vi "Audio Plugin UI Meas Ser1 - multichannel.vi"() -> ()   [LabVIEW 2021]
uses:
  <vilib>/PDM Acquisition Toolkit/shared/controls/i2s frame size.ctl
  <vilib>/PDM Acquisition Toolkit/host/Classes/Tasks/PDM Tasks/Controls/Acquisition Mode.ctl
  <vilib>/addons/_NISVFA/_Shared subVIs/Controls/svc_Window.ctl
  <vilib>/addons/_NISVFA/_Shared subVIs/Common/SVL Set dB Reference (N Ch - 1 Ref).vi
  <vilib>/addons/Sound and Vibration/svt_Level/SVL AC & DC Level (Time) (N Ch).vi
  <vilib>/addons/Sound and Vibration/svt_Single Tone Measurements/SVT Spurious Free Dynamic Range (Frequency) (1 Ch).vi
  <vilib>/addons/_NISVFA/_Shared subVIs/Common/SVL Set dB Reference (1 Ch).vi
  <vilib>/addons/Sound and Vibration/svt_Level/SVL AC & DC Level (Time) (1 Ch).vi
  <vilib>/addons/_NISVFA/_Spectrum Processing/SVFA Get Spectrum Subset.vi
  <vilib>/addons/_NISVFA/_Spectrum Processing/SVFA Get Spectrum Subset (Complex) (1 Ch).vi
  <vilib>/addons/_NISVFA/_Shared subVIs/Common/svc_Window Parameters.vi
  <vilib>/addons/_NISVFA/_Shared subVIs/Common/svc_Extract Single Tone Information (complex).vi
  <vilib>/addons/_NISVFA/_Shared subVIs/Common/svc_Check Frequency Range in Spectrum.vi
  <vilib>/addons/_NISVFA/_Spectrum Processing/SVFA Unit Conversion.vi
  <vilib>/addons/_NISVFA/_Spectrum Processing/SVFA Unit Conversion (Complex) (1 Ch).vi
  <vilib>/addons/_NISVFA/_Spectrum Processing/SVFA Spectrum Peak Search.vi
  <vilib>/addons/_NISVFA/_Spectrum Processing/SVFA Spectrum Peak Search (1 Ch).vi
  <vilib>/addons/_NISVFA/_Shared subVIs/Common/svc_Spectrum Units.vi
  <vilib>/addons/_NISVFA/_Shared subVIs/Common/SVL Set dB Reference (variant).vi
  <vilib>/addons/_NISVFA/_Shared subVIs/Common/svc_Get SV Channel Info.vi
  <vilib>/Analysis/baseanly.llb/Mean.vi
  <vilib>/Analysis/baseanly.llb/Mean (DBL).vi
  <vilib>/addons/_NISVFA/_Shared subVIs/Windowing/svfa_Scaled Time Domain Window (Array).vi
  <vilib>/addons/_NISVFA/_Shared subVIs/Common/svc_Build Unit Label for Frequency Range.vi
  <vilib>/addons/_NISVFA/_Spectrum Processing/SVFA Get Tone Amplitude and Phase (1 Ch).vi
  <vilib>/addons/_NISVFA/_Spectrum Processing/subVIs/svfa_Compute Complex Spectrum for Export.vi
  <vilib>/addons/_NISVFA/_Shared subVIs/Common/svc_Check Frequency Range in Bandwidth.vi
  <vilib>/addons/_NISVFA/_Shared subVIs/Common/svc_Convert Start and Stop to Start Index and Length.vi
  <vilib>/addons/_NISVFA/_Shared subVIs/Common/svc_Log View for Spectrum (1Ch).vi
  <vilib>/addons/_NISVFA/_Spectrum Processing/SVFA Unit Conversion (1 Ch).vi
  <vilib>/addons/_NISVFA/_Shared subVIs/Common/svc_Complex Datatype Defaults.vi
  <vilib>/addons/_NISVFA/_Spectrum Processing/subVIs/svfa_Spectrum Peak Search.vi
  <vilib>/addons/_NISVFA/_Shared subVIs/Common/svc_Format Value (DBL).vi
  <vilib>/addons/_NISVFA/_Shared subVIs/Common/svc_Get Weighting Enum and Labels.vi
  <vilib>/addons/_NISVFA/_Shared subVIs/Common/svc_Engineering Units to Unit Label.vi
  <vilib>/addons/_NISVFA/_Shared subVIs/Common/svc_Surround NonAlpha String with Parentheses.vi
  <vilib>/dlg_ctls.llb/Space Constant.vi
  <vilib>/addons/_NISVFA/_Shared subVIs/Common/svc_Unit Label to Engineering Units.vi
  <vilib>/addons/_NISVFA/_Spectrum Processing/subVIs/svfa_Spectrum Info Window to windowTd Type Def.vi
  <vilib>/Analysis/4window.llb/Force Window.vi
  <vilib>/Analysis/4window.llb/Force Window (DBL).vi
  <vilib>/Analysis/4window.llb/Exponential Window.vi
  <vilib>/Analysis/4window.llb/Exponential Window (DBL).vi
  <vilib>/addons/_NISVFA/_Spectrum Processing/subVIs/svfa_Window Frequency Response.vi
  <vilib>/addons/_NISVFA/_Spectrum Processing/subVIs/svfa_Window Frequency Response (double array).vi
  <vilib>/Analysis/baseanly.llb/Dot Product.vi
  <vilib>/Analysis/baseanly.llb/Complex Dot Product.vi
  <vilib>/addons/_NISVFA/_Shared subVIs/Common/svc_Unwrap Phase.vi
  <vilib>/addons/_NISVFA/_Shared subVIs/Common/svc_Convert Spectrum Array to dB.vi
  <vilib>/addons/_NISVFA/_Spectrum Processing/subVIs/svfa_Conversion Utility (spectrum info).vi
  <vilib>/addons/_NISVFA/_Spectrum Processing/subVIs/svfa_Peak Rough Search Indices.vi
  <vilib>/addons/_NISVFA/_Shared subVIs/Common/svc_Unit Label Lexical Class.vi
  <vilib>/addons/_NISVFA/_Spectrum Processing/subVIs/svfa_Rect Window Frequency Response.vi
  <vilib>/addons/_NISVFA/_Spectrum Processing/subVIs/svfa_Cosine Window Coefficients.vi
  <vilib>/addons/_NISVFA/_Spectrum Processing/subVIs/svfa_Peak to RMS to Peak2Peak.vi
  <vilib>/addons/_NISVFA/_Spectrum Processing/subVIs/svfa_Mag to Mag2.vi
  <vilib>/addons/_NISVFA/_Spectrum Processing/subVIs/svfa_Linear to dB.vi
  <vilib>/addons/_NISVFA/_Spectrum Processing/subVIs/svfa_dBrefA to dBrefB.vi
  <vilib>/addons/_NISVFA/_Spectrum Processing/subVIs/svfa_Spectrum to Spectral Density.vi
  <vilib>/PDM Acquisition Toolkit/host/API/Public/Create Tasks/Create I2S Input Task.vi
  <vilib>/PDM Acquisition Toolkit/host/API/Public/Configure/Timing/Configure Timing - I2S Input Slave.vi
  <vilib>/PDM Acquisition Toolkit/host/API/Public/Configure/PDM Channel/Configure Microphone Sensitivity FSPA - I2S Input Task.vi
  <vilib>/DAQmx/create/channels.llb/DAQmx Create Channel (AO-FuncGen).vi
  <vilib>/PDM Acquisition Toolkit/host/API/Public/Commit/Commit I2S Input Task.vi
  <vilib>/PDM Acquisition Toolkit/host/API/Public/Start/Start I2S Input Task.vi
  <vilib>/PDM Acquisition Toolkit/host/API/Public/Read/Read I2S Waveform.vi
  <vilib>/PDM Acquisition Toolkit/host/API/Public/Clear/Clear I2S Input Task.vi
  <vilib>/addons/Sound and Vibration/svt_Weighting/SVT Weighting Filter (N Ch).vi
  <vilib>/addons/_NISVFA/_Shared subVIs/Common/svc_Caller VI Returned in Error Source.vi
  <vilib>/addons/_NISVFA/_Shared subVIs/Common/svc_Get Window Info.vi
  <vilib>/Analysis/0measdsp.llb/Scaled Time Domain Window.vi
  <vilib>/Analysis/0measdsp.llb/Scaled Time Domain Window (DBL).vi
  <vilib>/Utility/error.llb/Error Cluster From Error Code.vi
  <vilib>/Analysis/baseanly.llb/Std Deviation and Variance.vi
  <vilib>/addons/Sound and Vibration/svt_Single Tone Measurements/SVT Gain (Time) (1 Ch).vi
  <vilib>/addons/Sound and Vibration/svt_Distortion/SVT SNR without Harmonics (Frequency) (1 Ch).vi
  <vilib>/addons/Sound and Vibration/svt_Single Tone Measurements/SVT Dynamic Range (Frequency) (1 Ch).vi
  <vilib>/addons/Sound and Vibration/svt_Distortion/subVIs/sv_Check Data Valid (Audio) (1 Ch).vi
  <vilib>/addons/_NISVFA/_Shared subVIs/Common/svc_Convert Frequency to Frequency String.vi
  <vilib>/Analysis/4window.llb/window parameters.vi
  <vilib>/Analysis/4window.llb/Window Properties.vi
  <vilib>/Analysis/4window.llb/Window Properties by Name.vi
  <vilib>/addons/_NISVFA/_Spectrum Processing/subVIs/svfa_Spectrum Peak Tone Search and Estimation (complex).vi
  <vilib>/measure/masignal.llb/Tones and Noise Waveform.vi
  <vilib>/addons/_NISVFA/_Shared subVIs/Common/svc_FFT with Window.vi
  <vilib>/Analysis/1siggen.llb/Square Wave.vi
  <vilib>/addons/_NISVFA/_Spectrum Processing/subVIs/svfa_Three Finger Peak Search.vi
  <vilib>/addons/Sound and Vibration/svt_Distortion/subVIs/sv_Peak View Amplitude (1 Ch).vi
  <vilib>/PDM Acquisition Toolkit/host/Classes/Tasks/PDM Tasks/PDM Task.lvclass
  <vilib>/PDM Acquisition Toolkit/host/API/PDM Acquisition Toolkit.lvlib
  <vilib>/addons/Sound and Vibration/svt_Single Tone Measurements/SoundVib_SingleTone.lvlib
  <vilib>/addons/Sound and Vibration/svt_Distortion/SoundVib_Distortion.lvlib
  <vilib>/PDM Acquisition Toolkit/shared/PDM Shared.lvlib
  <vilib>/addons/Sound and Vibration/svt_Weighting/SoundVib_ABCWeighting.lvlib
panel:
  in  "Array":string[](array[string])
  in  "weighting":u16(ring) items=["Linear", "A-weighting", "B-weighting", "C-weighting"]
  in  "Bits per Sample":u32=16 caption="BITS PER SAMPLE"
  in  "DUT full scale (V pk)":dbl=3.16 format="%.3p"
  out "error out":errorcluster
  out "Sampling Rate":dbl=192000.0 format="%#_6p"
  in  "I2S Data Latch at SCK Cycle":u8=50 caption="DATA LATCH AT SCK" format="%.0f%"
  out "MeasTable":string[][](table)
  in  "I2S Logic Level":enum16{"3.3 V", "1.8 V", "1.2 V"}(ring) caption="LOGIC LEVEL"
  in  "I2S Frame Size":enum16{"32bits", "64bits"}(ring)=enum."64bits" caption="FRAME SIZE"
  in  "I2S Number of Words":u32=19200 caption="NO OF WORDS"
  in  "I2S Word Length":u32=24 caption="WORD LENGTH"
  in  "I2S Clock Rate":u32=12288000 caption="CLOCK RATE"
  in  "THD Maximum Harmonic":u32=9 caption="MAX HARMONIC"
  in  "Measurement Band Stop":dbl=20000.0 caption="BAND STOP" format="%#_6pHz"
  in  "Measurement Band Start":dbl=20.0 caption="BAND START" format="%#_6pHz"
  in  "DSG amplitude":dbl=1.0 caption="AMPLITUDE" format="%#_6pV"
  in  "DSG frequency":dbl=1000.0 caption="FREQUENCY" format="%#_6pHz"
  in  "Mic sensitivity (FS/Pa)":dbl=0.34762 caption="MIC SENSITIVITY" format="%.3fFS/Pa"
  in  "I2S Channel List":string="PXI1Slot7\\I2Si 0" caption="CHANNEL LIST"
  out "MeasGraphs":enum32{"Time Domain", "Histogram", "DNL", "INL"}(tab)
  out "TimeDomain":waveform(dbl)[](graph) caption="AC"
  # "Can we hard code Sensitivity? \nAdd weighting filter option from SV toolkit"
  # "Analog Source"
  # "Measurement"
  # "I2S Setting"
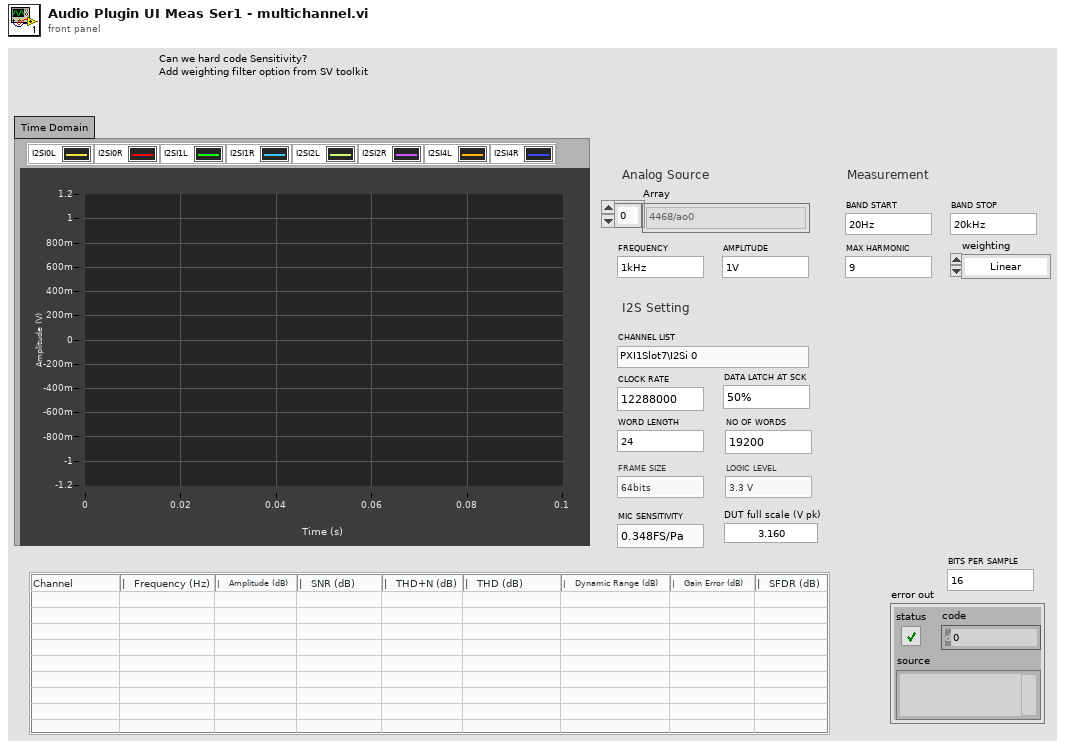
[diagram p1: front panel]
types:
  T1 = cluster{"band start (Hz)":dbl, "band stop (Hz)":dbl}
  T2 = typedef "PDM Shared.lvlib/i2s frame size.ctl" = enum16{"32bits", "64bits"}
  T3 = cluster{"frequency range":cluster{"band start (Hz)":dbl, "band stop (Hz)":dbl}, "THD maximum harmonic":i32, "amplitude":dbl, "frequency (Hz)":dbl, "microphone sensitivity (FS/Pa)":dbl, "number of words":i32, "channel list":string, "logic level":enum16{"3.3 V", "1.8 V", "1.2 V"}, "I2S serial clock rate 2":u32, "frame size":T2, "word length":u32, "Data Latch at SCK cycle":u8, "Playback .WAV File?":bool, "Record .WAV File?":bool, "Record wave file path":path, "Playback .WAV file path":path, "number of channels":i32, "DUT full scale (V pk)":dbl, "output channel":tag[]}
  T4 = typedef "PDM Acquisition Class Library.lvlib/PDM Task.lvclass/Acquisition Mode.ctl" = enum16{"Finite", "Continuous"}
  T5 = cluster{"gain units":enum16{"dB", "linear ratio"}, "detected fundamental amplitude units":enum16{"EU rms", "EU peak", "EU peak-peak"}}
  T6 = cluster{"SNR units":enum16{"dB", "linear ratio", "%"}, "detected fundamental amplitude units":enum16{"EU rms", "EU peak", "EU peak-peak"}}
  T7 = typedef "PDM Acquisition Class Library.lvlib/I2S Input Task.lvclass/DVR I2S Input Task.ctl" = refnum<data-value>
  T8 = typedef "svc_Window.ctl" = u32
  T9 = typedef "svc_Spectrum Info.ctl" = cluster{"channel name":string, "description":string, "x-axis units":T10, "spectral info":cluster{"spectrum type":T11, "linear/dB":enum16{"linear", "dB"}, "window":u16, "window size":i32, "FFT size":i32}, "engineering units":T12, "custom label":string, "dB reference [EU]":dbl, "peak units":enum16{"rms", "peak", "peak-peak"}, "weighting filter":T13, "spectral density?":bool, "unit label":string, "spectrum skewed?":bool, "complimentary spectrum units":T14}
  T10 = typedef "svc_X-Axis Units.ctl" = u16
  T11 = typedef "svc_Spectrum Type.ctl" = enum16{"FFT Spectrum [complex]", "Amplitude [Magnitude]", "Power [Magnitude^2]", "Cross Spectrum [complex]", "Frequency Response [Complex]"}
  T12 = typedef "svc_Engineering Units Text Ring.ctl" = u16
  T13 = typedef "svc_Weighting Filter Text Ring.ctl" = u16
  T14 = typedef "svc_Complimentary Spectrum Units.ctl" = enum16{"none", "radians", "degrees", "cycles", "imaginary"}
  T15 = cluster{"complex spectrum response":cluster{"f0":dbl, "df":dbl, "complex spectrum":cdb[]}, "spectrum info":T9}
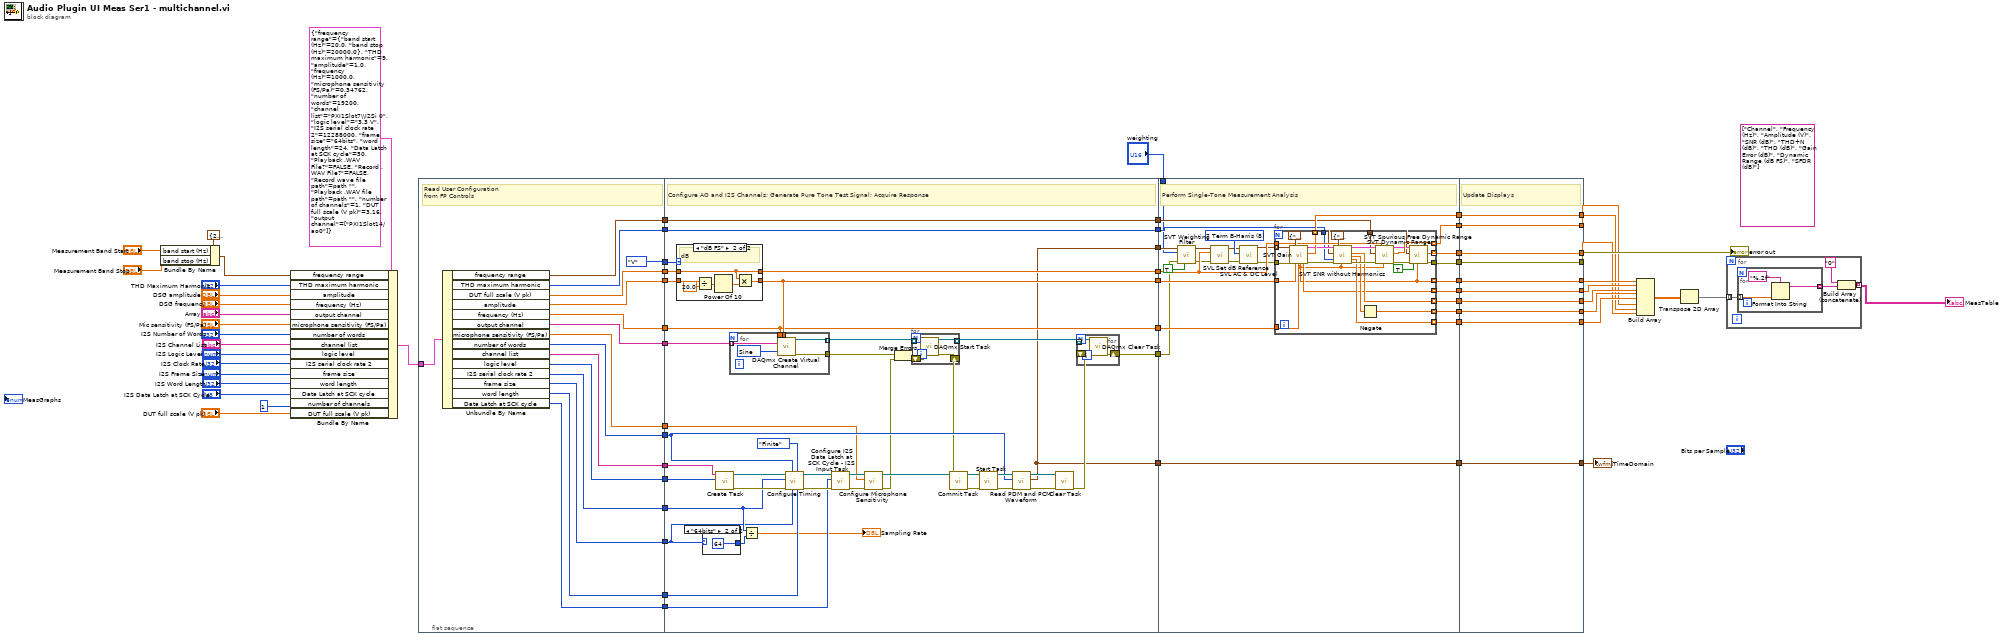
[diagram p0: block diagram]
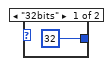
[diagram p2: hidden frame]
diagram:
  (unwired) string[] ["Channel", "Frequency (Hz)", "Amplitude (V)", "SNR (dB)", "THD+N (dB)", "THD (dB)", "Gain Error (dB)", "Dynamic Range (dB FS)", "SFDR (dB)"] ("MeasTable")
  n1 = Bundle By Name(cluster=T1 {"band start (Hz)"=20.0, "band stop (Hz)"=20000.0} ("frequency range"), "band start (Hz)"="Measurement Band Start", "band stop (Hz)"="Measurement Band Stop") -> (w33:T1)
  n2 = Bundle By Name(cluster=T3 {"frequency range"={"band start (Hz)"=20.0, "band stop (Hz)"=20000.0}, "THD maximum harmonic"=9, "amplitude"=1.0, "frequency (Hz)"=1000.0, "microphone sensitivity (FS/Pa)"=0.34762, "number of words"=19200, "channel list"="PXI1Slot7\\I2Si 0", "logic level"=enum."3.3 V", "I2S serial clock rate 2"=12288000, "frame size"=enum."64bits", "word length"=24, "Data Latch at SCK cycle"=50, "Playback .WAV File?"=FALSE, "Record .WAV File?"=FALSE, "Record wave file path"=path "", "Playback .WAV file path"=path "", "number of channels"=1, "DUT full scale (V pk)"=3.16, "output channel"=["PXI1Slot14/ao0"]}, "frequency range"=w33, "THD maximum harmonic"="THD Maximum Harmonic", "amplitude"="DSG amplitude", "frequency (Hz)"="DSG frequency", "output channel"="Array", "microphone sensitivity (FS/Pa)"="Mic sensitivity (FS/Pa)", "number of words"="I2S Number of Words", "channel list"="I2S Channel List", "logic level"="I2S Logic Level", "I2S serial clock rate 2"="I2S Clock Rate", "frame size"="I2S Frame Size", "word length"="I2S Word Length", "Data Latch at SCK cycle"="I2S Data Latch at SCK Cycle", "number of channels"=1, "DUT full scale (V pk)"="DUT full scale (V pk)") -> (w20:T3)
  n3 = flat-sequence {
    tunnel: [w80] -> w67
    tunnel: [w77] -> w66
    tunnel: [w76] -> w65
    tunnel: [w79] -> w64
    tunnel: [w78] -> w63
    tunnel: [enum16{"V", "dB FS"}."V" ("amplitude units")] -> w62
    tunnel: [w71] -> w61
    tunnel: [w72] -> w60
    tunnel: [w68] -> w59
    tunnel: [w74] -> w58
    tunnel: [w69] -> w57
    tunnel: [w70] -> w56
    tunnel: [w73] -> w55
    tunnel: [w75] -> w39
    tunnel: w20 -> [w82]
    tunnel: [w81] -> w19
    tunnel: w67 -> [w121]
    tunnel: w66 -> [w114]
    tunnel: w65 -> [w119]
    tunnel: w64 -> [w124]
    tunnel: w63 -> [w123]
    tunnel: w62 -> [w120]
    tunnel: [w125] -> w54
    tunnel: [w122] -> w53
    tunnel: [w121] -> w52
    tunnel: [w118] -> w51
    tunnel: [w114] -> w50
    tunnel: [w84] -> w49
    tunnel: [w112] -> w48
    tunnel: w61 -> [w96]
    tunnel: w60 -> [w95]
    tunnel: w59 -> [w94]
    tunnel: w58 -> [w93]
    tunnel: w57 -> [w92]
    tunnel: w56 -> [w91]
    tunnel: w55 -> [w90]
    tunnel: w39 -> [w85]
    tunnel: w19 -> [w125]
    tunnel: [w84] -> w15
    tunnel: [w169] -> w47
    tunnel: [w168] -> w46
    tunnel: [w159] -> w45
    tunnel: [w167] -> w44
    tunnel: [w166] -> w43
    tunnel: [w165] -> w42
    tunnel: [w164] -> w41
    tunnel: [w158] -> w40
    tunnel: w54 -> [w157]
    tunnel: w53 -> [w171]
    tunnel: w52 -> [w162]
    tunnel: w51 -> [w170]
    tunnel: w50 -> [w163]
    tunnel: w49 -> [w155]
    tunnel: w48 -> [w153]
    tunnel: [w160] -> w16
    tunnel: w15 -> [w160]
    tunnel: [w156] -> w14
    tunnel: "weighting" -> [w151]
    tunnel: w47 -> [w203]
    tunnel: w46 -> [w202]
    tunnel: w45 -> [w210]
    tunnel: w44 -> [w204]
    tunnel: w43 -> [w205]
    tunnel: w42 -> [w206]
    tunnel: w41 -> [w207]
    tunnel: w40 -> [w208]
    tunnel: [w210] -> w38
    tunnel: [w209] -> w17
    tunnel: w16 -> [w209]
    tunnel: w14 -> [w201]
    tunnel: [w208] -> w13
    tunnel: [w207] -> w12
    tunnel: [w206] -> w11
    tunnel: [w205] -> w10
    tunnel: [w204] -> w9
    tunnel: [w203] -> w8
    tunnel: [w202] -> w7
    tunnel: [w201] -> w6
    frame #0 {
      # "Read User Configuration\nfrom FP Controls"
      n4 = Unbundle By Name(w82) -> ("frequency range"=w81:T1, "THD maximum harmonic"=w80:i32, "DUT full scale (V pk)"=w79:dbl, "amplitude"=w78:dbl, "frequency (Hz)"=w77:dbl, "output channel"=w76:tag[], "microphone sensitivity (FS/Pa)"=w75:dbl, "number of words"=w74:i32, "channel list"=w73:string, "logic level"=w72:enum16{"3.3 V", "1.8 V", "1.2 V"}, "I2S serial clock rate 2"=w71:u32, "frame size"=w70:T2, "word length"=w69:u32, "Data Latch at SCK cycle"=w68:u8)
    }
    frame #1 {
      # "Configure AO and I2S Channels; Generate Pure Tone Test Signal; Acquire Response"
      n5 = case shown="\"dB FS\"" w120 {
        tunnel: [w142 w144] -> w118
        tunnel: w123 -> [w142 w148]
        tunnel: w124 -> [w141 w143]
        tunnel: [w141 w143] -> w122
        frame Default {
          # "V"
        }
        frame "dB FS" {
          # "dB"
          n6 = Divide(x=w148, y=20.0) -> (x/y=w146:dbl)
          n7 = Power Of 10(x=w146) -> (10^x=w145:dbl)
          n8 = Multiply(x=w143, y=w145) -> (x*y=w144:dbl)
        }
      }
      n9 = case shown="\"64bits\"" w91 {
        tunnel: [u8 32 ("frame size") u8 64 ("frame size")] -> w100
        frame "32bits" {
        }
        frame "64bits" {
        }
      }
      n10 = call-poly <vilib>:"Create Task.vi"("logic level"=w95, "channel list"=w90) -> ("error out"=w106:errorcluster, "I2S input task out"=w105:T7)  [unwired: 8 in]
      n11 = for {
        tunnel: w119 -> [w138] mode=indexing
        tunnel: w118 -> [w137]
        tunnel: [w136] -> w117
        tunnel: [w135] -> w115 mode=indexing
        tunnel: w114 -> [w134]
        w133 = 14751 items=["Sine"=14751, "Triangle"=14752, "Square"=14753, "Sawtooth"=14754] ("type")
        n12 = call-poly <vilib>:"DAQmx Create Virtual Channel.vi"("frequency"=w134, "amplitude"=w137, "physical channels"=w138, "type"=w133) -> ("task out"=w135:refnum<k21>, "error out"=w136:errorcluster)  [unwired: 10 in]
      }
      n13 = Divide(x=w96, y=w100) -> (x/y=→"Sampling Rate":dbl)
      n14 = call-poly <vilib>:"Configure Timing.vi"("word length"=w92, "acquisition mode"=Acquisition_Mode."Finite", "frame size"=w91, "number of words"=w93, "error in"=w106, "I2S serial clock rate"=w96, "I2S input task in"=w105) -> ("error out"=w104:errorcluster, "I2S input task out"=w101:T7)  [unwired: 3 in]
      n15 = call <vilib>:"Configure I2S Data Latch at SCK Cycle - I2S Input Task.vi"("error in"=w104, "data latch at SCK cycle"=w94, "I2S input task in"=w101) -> ("error out"=w103:errorcluster, "I2S input task out"=w102:T7)  [unwired: 7 in]
      n16 = call-poly <vilib>:"Configure Microphone Sensitivity.vi"("error in"=w103, "microphone sensitivity (FS/Pa)"=w85, "I2S input task in"=w102) -> ("error out"=w89:errorcluster, "I2S input task out"=w99:T7)  [unwired: 7 in]
      n17 = Merge Errors(w117, w89) -> (w116:errorcluster)
      n18 = for {
        tunnel: w115 -> [w131] mode=indexing
        tunnel: [w130] -> w113 mode=indexing
        shift-right: [w129] -> w88
        shift-left: w116 -> [w132]
        n19 = call <vilib>:"DAQmx Start Task.vi"("task/channels in"=w131, "error in"=w132) -> ("task out"=w130:refnum<k21>, "error out"=w129:errorcluster)  [unwired: 12 in]
      }
      n20 = call-poly <vilib>:"Commit Task.vi"("error in"=w88, "I2S input task in"=w99) -> ("error out"=w98:errorcluster, "I2S input task out"=w97:T7)  [unwired: 8 in]
      n21 = call-poly <vilib>:"Start Task.vi"("error in"=w98, "I2S input task in"=w97) -> ("error out"=w110:errorcluster, "I2S input task out"=w109:T7)  [unwired: 8 in]
      n22 = call-poly <vilib>:"Read PDM and PCM Waveform.vi"("error in"=w110, "words per channel"=w93, "I2S input task in"=w109) -> ("error out"=w108:errorcluster, "I2S waveforms"=w84:waveform(dbl)[], "I2S input task out"=w107:T7)  [unwired: 4 in, 2 out]
      n23 = call-poly <vilib>:"Clear Task.vi"("error in"=w108, "I2S input task in"=w107) -> ("error out"=w87:errorcluster)  [unwired: 9 in]
      n24 = for {
        tunnel: w113 -> [w128] mode=indexing
        shift-right: [w127] -> w112
        shift-left: w87 -> [w126]
        n25 = call <vilib>:"DAQmx Clear Task.vi"("task in"=w128, "error in"=w126) -> ("error out"=w127:errorcluster)  [unwired: 13 in]
      }
    }
    frame #2 {
      w174 = T8 8 items=["None"=0, "Hanning"=1, "Hamming"=2, "Blackman-Harris"=3, "Exact Blackman"=4, "Blackman"=5, "Flat Top"=6, "4 Term B-Harris "=7, "7 Term B-Harris"=8, "Low Sidelobe"=9, "Force"=64, "Exponential"=65, "Blackman Nuttall"=11, "Triangle"=30, "Bartlett-Hanning"=31, "Bohman"=32, "Parzen"=33, "Welch"=34, "Kaiser"=60, "Dolph-Chebyshev"=61, "Gaussian"=62] ("window")
      # "Perform Single-Tone Measurement Analysis"
      n26 = call-poly <vilib>:"SVT Weighting Filter.vi"("reset filter (F)"=TRUE, "error in (no error)"=w153, "weighting"=w151, "scaled signals [EU]"=w155) -> ("error out"=w152:errorcluster, "weighted signals [EU]"=w154:waveform(dbl)[])  [unwired: 5 in]
      n27 = call-poly <vilib>:"SVL Set dB Reference.vi"("error in (no error)"=w152, "dB reference [EU]"=w171, "scaled signals in [EU]"=w154) -> ("error out"=w173:errorcluster, "scaled signals out [EU]"=w172:waveform(dbl)[])  [unwired: 7 in]
      n28 = call-poly <vilib>:"SVL AC & DC Level.vi"("scaled signals in [EU]"=w172, "window"=w174, "error in (no error)"=w173) -> ("AC signals [EU]"=w149:waveform(dbl)[], "error out"=w161:errorcluster)  [unwired: 11 in, 4 out]
      n29 = for {
        tunnel: w170 -> [w193]
        tunnel: [w192] -> w169 mode=indexing
        tunnel: [w190] -> w167 mode=indexing
        tunnel: [w189] -> w166 mode=indexing
        tunnel: [w188] -> w165 mode=indexing
        tunnel: [w187] -> w164 mode=indexing
        tunnel: w163 -> [w186]
        tunnel: w162 -> [w184]
        tunnel: [w179] -> w158 mode=indexing
        tunnel: w157 -> [w178]
        tunnel: [w176] -> w156 mode=indexing
        tunnel: w149 -> [w175] mode=indexing
        tunnel: w171 -> [w194]
        tunnel: [w191] -> w168 mode=indexing
        tunnel: w161 -> [w183]
        tunnel: [w180] -> w159
        n30 = call-poly <vilib>:"SVT Gain.vi"("scaled signal [EU]"=w175, "error in (no error)"=w183, "desired units"=T5 {"gain units"=enum."dB", "detected fundamental amplitude units"=enum."EU peak"}, "amplitude [EU peak]"=w193, "expected fundamental frequency [Hz]"=w186) -> ("detected fundamental\nfrequency [Hz]"=w179:dbl, "detected fundamental\namplitude"=w187:dbl, "complex spectrum"=w185:T15, "gain"=w192:dbl, "error out"=w200:errorcluster)  [unwired: 9 in, 1 out]
        n31 = call-poly <vilib>:"SVT SNR without Harmonics.vi"("complex spectrum"=w185, "frequency range"=w178, "maximum harmonic"=w184, "error in (no error)"=w200, "desired units"=T6 {"SNR units"=enum."dB", "detected fundamental amplitude units"=enum."EU rms"}, "expected fundamental frequency [Hz]"=w179) -> ("complex spectrum"=w198:T15, "SNR (without harmonics)"=w188:dbl, "SINAD"=w197:dbl, "THD"=w190:dbl, "error out"=w199:errorcluster)  [unwired: 6 in, 3 out]
        n32 = Negate(x=w197) -> (-x=w189:dbl)
        n33 = call-poly <vilib>:"SVT Dynamic Range.vi"("complex spectrum"=w198, "frequency range"=w178, "error in (no error)"=w199, "full scale amplitude [EU peak]"=w194, "expected fundamental\nfrequency [Hz]"=w179) -> ("dup complex spectrum"=w182:T15, "dynamic range"=w191:dbl, "error out"=w181:errorcluster)  [unwired: 9 in, 3 out]
        n34 = call-poly <vilib>:"SVT Spurious Free Dynamic Range.vi"("complex spectrum"=w182, "frequency range"=w178, "error in (no error)"=w181, "exclude harmonics"=TRUE, "expected fundamental\nfrequency [Hz]"=w179) -> ("spurious free dynamic range"=w176:dbl, "error out"=w180:errorcluster)  [unwired: 7 in, 6 out]
      }
    }
    frame #3 {
      # "Update Displays"
    }
  }
  n35 = Build Array(w13, w12, w11, w10, w9, w8, w7, w6) -> (w5:dbl[][])
  n36 = Transpose 2D Array(2D array=w5) -> (transposed array=w3:dbl[][])
  n37 = for {
    tunnel: w3 -> [w214] mode=indexing
    tunnel: [w212] -> w2 mode=indexing
    n38 = for {
      tunnel: w214 -> [w217] mode=indexing
      tunnel: [w215] -> w213 mode=indexing
      n39 = Format Into String(format string="%.2f", w217) -> (resulting string=w215:string)  [unwired: 2 in, 1 out]
    }
    n40 = Build Array (concatenate)("0" ("format string"), w213) -> (w212:string[])
  }
  "MeasTable" <- w2
  "error out" <- w38
  "TimeDomain" <- w17
